vi "mod_Extract Burst.vi"(0 "Complex Waveform":cluster{"t0":dbl, "dt":dbl, "Y":cdb[]}, 5 "Triggers Found":cluster{"Start Index":dbl, "Stop Index":dbl}[](array[cluster]), 7 "Trigger Number to Extract(1st,2nd ..)":i32, 9 "Padding at beginning and end":i32, 11 "error in (no error)":errorcluster) -> (4 "Extracted Burst":cluster{"t0":dbl, "dt":dbl, "Y":cdb[]}, 15 "error out":errorcluster)   [LabVIEW 2020, in "niDMT.lvlib"]
uses:
  <vilib>/addons/Modulation/niDMT.lvlib
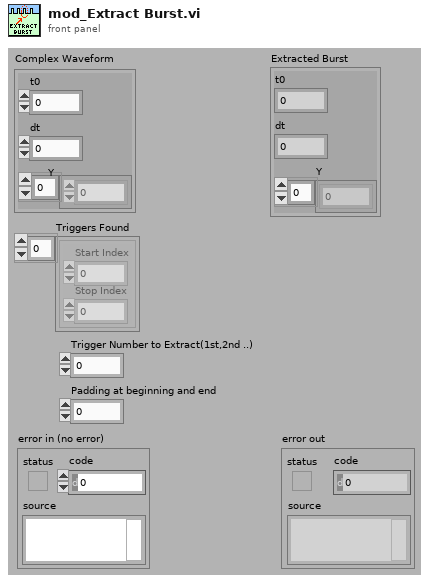
[diagram p1: front panel]
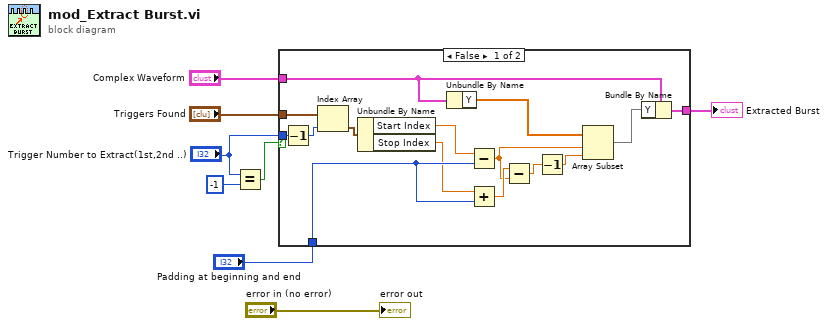
[diagram p0: block diagram]
diagram:
  n1 = Equal?(x="Trigger Number to Extract(1st,2nd ..)", y=-1) -> (x = y?=w3:bool)
  n2 = case shown="False" w3 {
    tunnel: "Triggers Found" -> [w23 _]
    tunnel: "Trigger Number to Extract(1st,2nd ..)" -> [w22 _]
    tunnel: "Complex Waveform" -> [w16 w24]
    tunnel: [w14 w24] -> w6
    tunnel: "Padding at beginning and end" -> [w13 _]
    frame False {
      n3 = Decrement(x=w22) -> (x-1=w21:i32)
      n4 = Index Array(array=w23, index=w21) -> (element=w20:cluster{"Start Index":dbl, "Stop Index":dbl})
      n5 = Unbundle By Name(w20) -> ("Start Index"=w10:dbl, "Stop Index"=w12:dbl)
      n6 = Unbundle By Name(w16) -> ("Y"=w19:cdb[])
      n7 = Subtract(x=w10, y=w13) -> (x-y=w9:dbl)
      n8 = Add(x=w12, y=w13) -> (x+y=w11:dbl)
      n9 = Subtract(x=w11, y=w9) -> (x-y=w18:dbl)
      n10 = Decrement(x=w18) -> (x-1=w17:dbl)
      n11 = Array Subset(array=w19, index=w9, length=w17) -> (w15:cdb[])
      n12 = Bundle By Name(cluster=w16, "Y"=w15) -> (w14:cluster{"t0":dbl, "dt":dbl, "Y":cdb[]})
    }
    frame True {
    }
  }
  "Extracted Burst" <- w6
  "error out" <- "error in (no error)"
